vi "Find Widest Flat Top.vi"(0 "Data In":dbl[](array[numeric])) -> (1 "start":i32, 2 "end":i32, 3 "width":i32, 4 "amplitude":dbl)   [LabVIEW 2012]
panel:
  out "data plot":dbl[](graph)
  # "*ignores flat tops at the BOTH ends of array*"
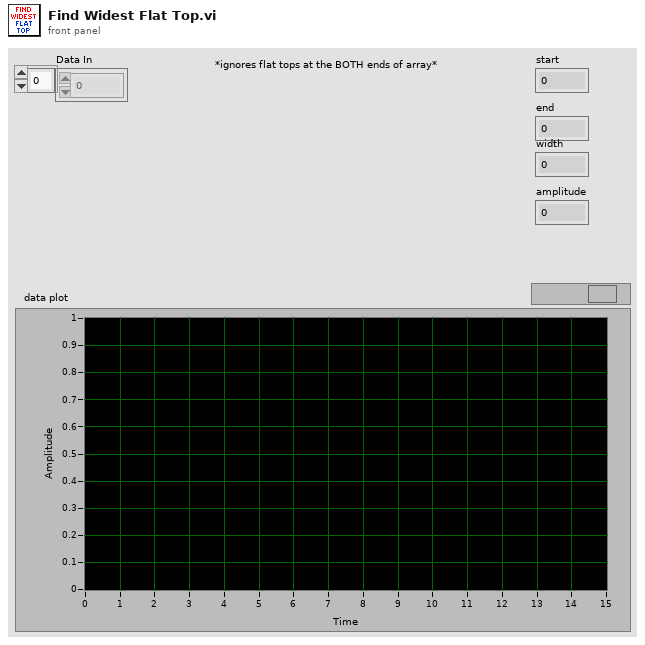
[diagram p1: front panel]
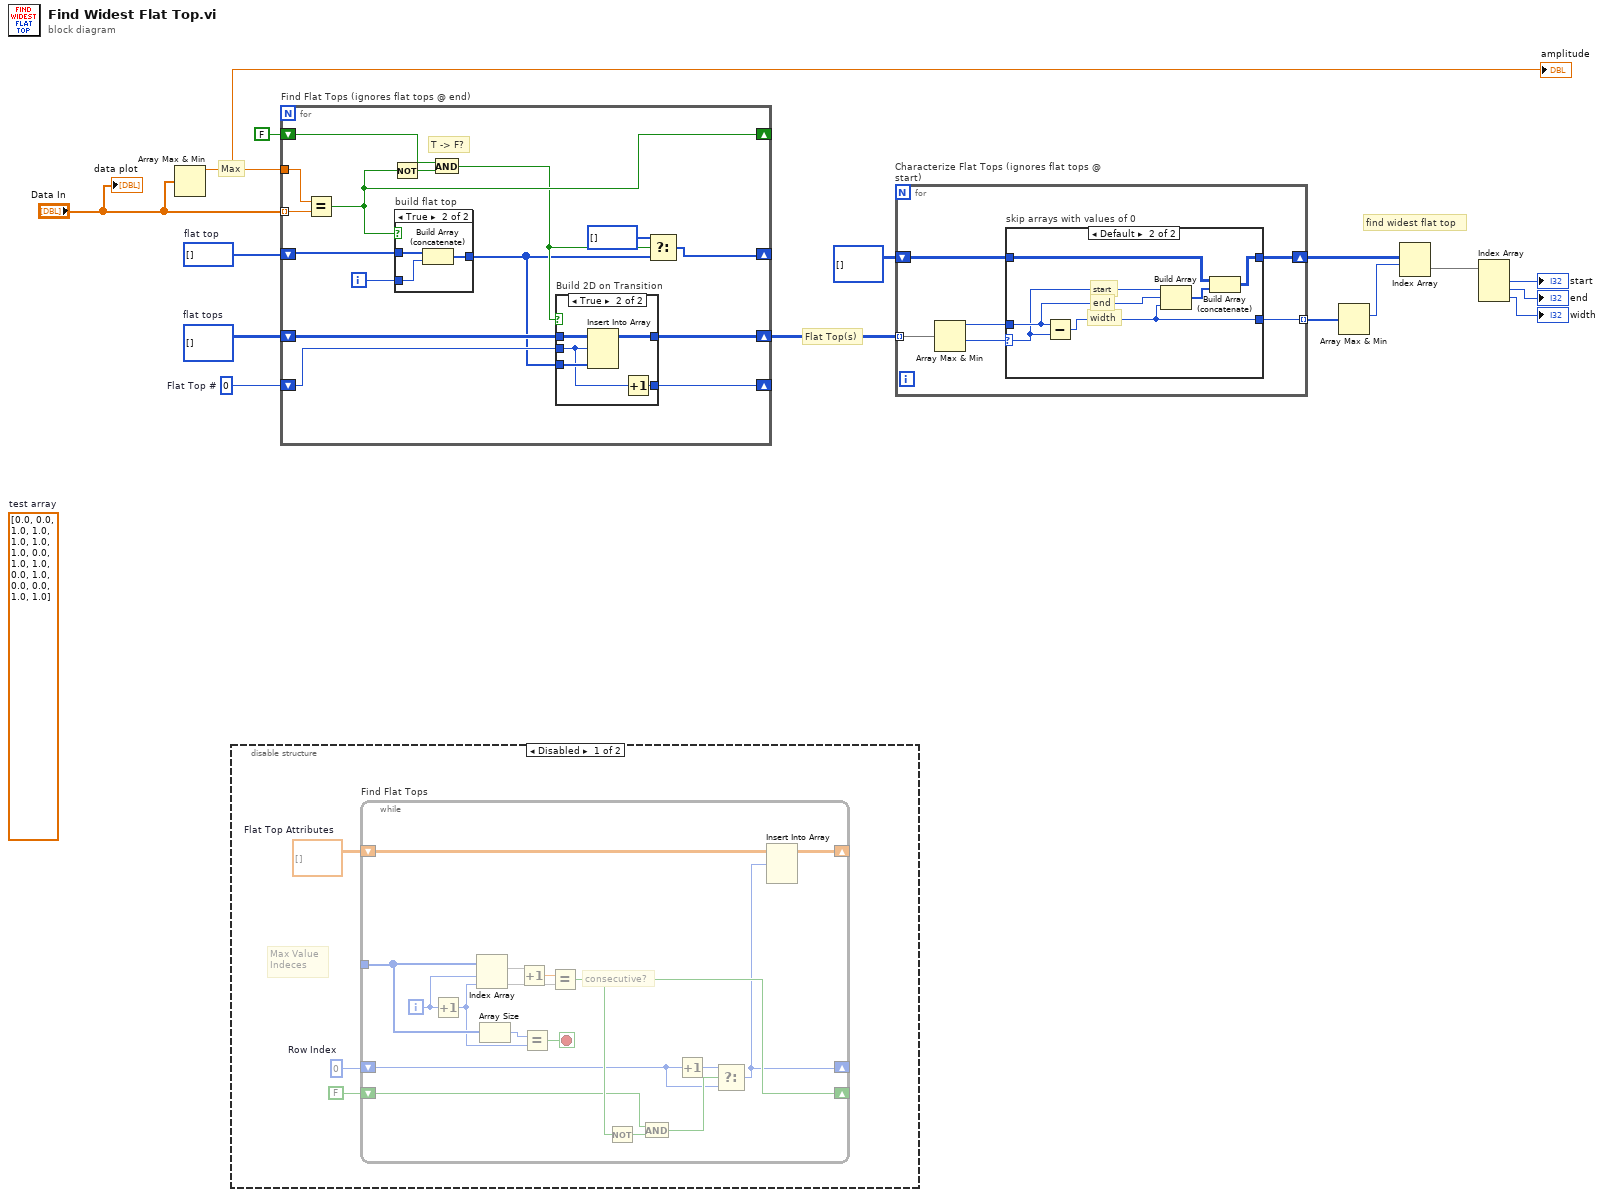
[diagram p0: block diagram]
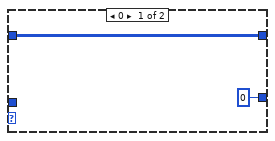
[diagram p2: hidden frame]
diagram:
  w11 = 0  # Flat Top #
  w13 = i32[][] []  # flat tops
  w14 = i32[] []  # flat top
  (unwired) dbl[] [0.0, 0.0, 1.0, 1.0, 1.0, 1.0, 1.0, 0.0, 1.0, 1.0, 0.0, 1.0, 0.0, 0.0, 1.0, 1.0]  # test array
  # "find widest flat top"
  # "Flat Top(s)"
  # "Max"
  n1 = Array Max & Min(array="Data In") -> (max value=w15:dbl)  [unwired: 3 out]
  "amplitude" <- w15
  n2 = disable-structure shown="Disabled" {
    frame Disabled {
      w17 = 0  # Row Index
      w18 = dbl[][] []  # Flat Top Attributes
      # "Max Value \nIndeces"
      n3 = while "Find Flat Tops" {
        tunnel: _ -> [w32]
        shift-right: [w21] -> _
        shift-left: w17 -> [w24]
        shift-right: [w22] -> _
        shift-left: w18 -> [w23]
        shift-right: [w27] -> _
        shift-left: FALSE -> [w19]
        i -> [w35]
        stop <- w33 stop-if-true
        # "consecutive?"
        n4 = Increment(x=w35) -> (x+1=w31:i32)
        n5 = Index Array(array=w32, index #1=w35, index #2=w31) -> (element #1=w20, element #2=w30)
        n6 = Array Size(array=w32) -> (size(s)=w34:i32)
        n7 = Increment(x=w20) -> (x+1=w29:dbl)
        n8 = Equal?(x=w34, y=w31) -> (x = y?=w33:bool)
        n9 = Equal?(x=w29, y=w30) -> (x = y?=w27:bool)
        n10 = Not(x=w27) -> (.not. x?=w28:bool)
        n11 = And(x=w19, y=w28) -> (x .and. y?=w26:bool)
        n12 = Increment(x=w24) -> (x+1=w25:i32)
        n13 = Select(t=w25, s=w26, f=w24) -> (s? t:f=w21:i32)
        n14 = Insert Into Array(array=w23, index (row)=w21) -> (w22:dbl[][])  [unwired: 2 in]
      }
    }
    frame Enabled {
    }
  }
  n15 = for "Find Flat Tops (ignores flat tops @ end)" {
    tunnel: w15 -> [w50]
    tunnel: "Data In" -> [w49] mode=indexing
    shift-right: [w36] -> _
    shift-left: w14 -> [w48]
    shift-right: [w40] -> _
    shift-left: FALSE ("x = y?") -> [w45]
    shift-right: [w42] -> _
    shift-left: w11 -> [w43]
    shift-right: [w41] -> w10
    shift-left: w13 -> [w46]
    i -> [w47]
    # "T -> F?"
    n16 = Equal?(x=w50, y=w49) -> (x = y?=w40:bool)
    n17 = Not(x=w40) -> (.not. x?=w44:bool)
    n18 = case "build flat top" shown="True" w40 {
      tunnel: w48 -> [w58 w61]
      tunnel: w47 -> [_ w60]
      tunnel: [w58 w59] -> w38
      frame False {
      }
      frame True {
        n19 = Build Array (concatenate)(w61, w60) -> (w59:i32[])
      }
    }
    n20 = And(x=w45, y=w44) -> (x .and. y?=w39:bool)
    n21 = case "Build 2D on Transition" shown="True" w39 {
      tunnel: w46 -> [w51 w57]
      tunnel: w38 -> [_ w56]
      tunnel: w43 -> [w52 w55]
      tunnel: [w52 w54] -> w42
      tunnel: [w51 w53] -> w41
      frame False {
      }
      frame True {
        n22 = Insert Into Array(array=w57, index (row)=w55, new element=w56) -> (w53:i32[][])  [unwired: 1 in]
        n23 = Increment(x=w55) -> (x+1=w54:i32)
      }
    }
    n24 = Select(t=i32[] [] ("flat top"), s=w39, f=w38) -> (s? t:f=w36:i32[])
  }
  n25 = for "Characterize Flat Tops (ignores flat tops @ start)" {
    tunnel: w10 -> [w67] mode=indexing
    shift-right: [w64] -> w8
    shift-left: i32[][] [] -> [w65]
    tunnel: [w63] -> w7 mode=indexing
    n26 = Array Max & Min(array=w67) -> (max value=w66:i32, min value=w62:i32)  [unwired: 2 out]
    n27 = case "skip arrays with values of 0" shown="Default" w62 {
      selector: w62 -> [_ w71]
      tunnel: w66 -> [_ w75]
      tunnel: w65 -> [w69 w74]
      tunnel: [w69 w72] -> w64
      tunnel: [0 w70] -> w63
      frame 0 {
      }
      frame Default {
        # "width"
        # "end"
        # "start"
        n28 = Subtract(x=w75, y=w71) -> (x-y=w70:i32)
        n29 = Build Array(w71, w75, w70) -> (w73:i32[])
        n30 = Build Array (concatenate)(w74, w73) -> (w72:i32[][])
      }
    }
  }
  n31 = Array Max & Min(array=w7) -> (max index (indices)=w6:i32)  [unwired: 3 out]
  n32 = Index Array(array=w8, index (row)=w6) -> (element=w5:i32[])  [unwired: 1 in]
  n33 = Index Array(array=w5) -> (element #1=→"start":i32, element #2=→"end":i32, element #3=→"width":i32)  [unwired: 3 in]
  "data plot" <- "Data In"
